vi "Prediction Back.vi"(8 "error in (no error)":errorcluster, 11 "Measurement in":refnum<class "Measurement.lvclass">) -> (0 "error out":errorcluster, 2 "Numeric":i64, 3 "Measurement out":refnum<class "Measurement.lvclass">)   [LabVIEW 2020, in "Measurement.lvclass"]
uses:
  Measurement.lvclass
  Measurement.lvclass/Measurement.ctl
panel:
  out "Array":i64[](array[numeric])
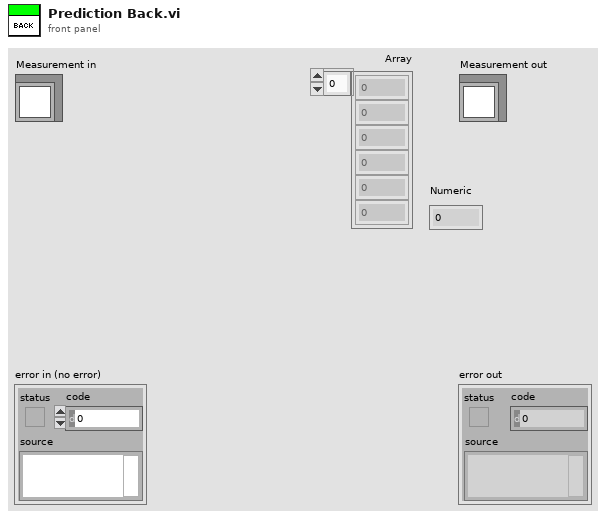
[diagram p1: front panel]
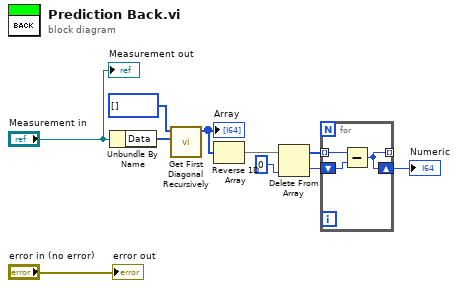
[diagram p0: block diagram]
diagram:
  n1 = Unbundle By Name("Measurement in") -> ("Data"=w8:i64[])
  n2 = call "Get First Diagonal Recursively.vi"("Data"=w8, "Result"=i64[] []) -> ("Array"=w6:i64[])  [unwired: 9 in]
  "Array" <- w6
  n3 = Reverse 1D Array(array=w6) -> (reversed array=w3:i64[])
  n4 = Delete From Array(array=w3, index=0) -> (deleted portion=w2:i64, array with subset deleted=w1:i64[])  [unwired: 1 in]
  n5 = for {
    tunnel: w1 -> [w12] mode=indexing
    shift-right: [w11] -> w5
    shift-left: w2 -> [w13]
    tunnel: [w11] -> _ mode=indexing
    n6 = Subtract(x=w12, y=w13) -> (x-y=w11:i64)
  }
  "Numeric" <- w5
  "error out" <- "error in (no error)"
  "Measurement out" <- "Measurement in"
